vi "MC_Debugging_CreateWireDescription.vi"(6 "End of Interpreted Statement?":bool, 7 "First Error Wire?":bool, 8 "UID?":bool, 9 "Text of Line":string, 10 "Breakpoint Line Numbers":i32[](array[numeric]), 11 "Variable Wire Info":T1) -> (3 "Wire Description":string)   [LabVIEW 2021]
uses:
  <vilib>/imath/engines/lvmath2/MathScriptCompiler/Debugging/MC_Debugging_VariableWireInfo.ctl
  <vilib>/imath/engines/lvmath2/MathScriptCompiler/Debugging/NIMS_Debugging_VariablesCluster.ctl
  <vilib>/imath/engines/lvmath2/RunTimeEngine/Debugging/MC_Debugging_ColVectorInfo.ctl
  <vilib>/imath/engines/lvmath2/RunTimeEngine/Debugging/MC_Debugging_WireData.ctl
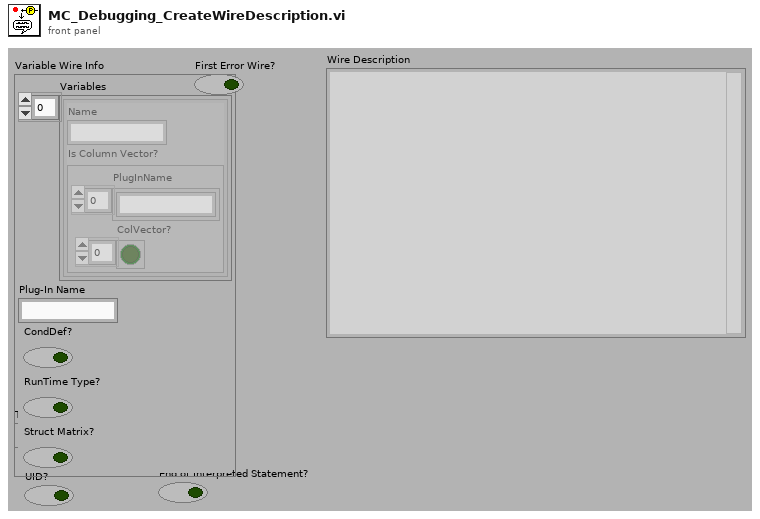
[diagram p1: front panel]
types:
  T1 = typedef "MC_Debugging_VariableWireInfo.ctl" = cluster{"Variables":T2[], "Plug-In Name":string, "CondDef?":bool, "RunTime Type?":bool, "Struct Matrix?":bool}
  T2 = typedef "NIMS_Debugging_VariablesCluster.ctl" = cluster{"Name":string, "Is Column Vector?":T3}
  T3 = typedef "MC_Debugging_ColVectorInfo.ctl" = cluster{"PlugInName":string[], "ColVector?":bool[]}
  T4 = typedef "MC_Debugging_WireData.ctl" = cluster{"Breakpoint Line Numbers":i32[], "Text of Line":string, "UID?":bool, "End of Interpreted Statement?":bool, "Variable Wire Info":T1, "First Error Wire?":bool}
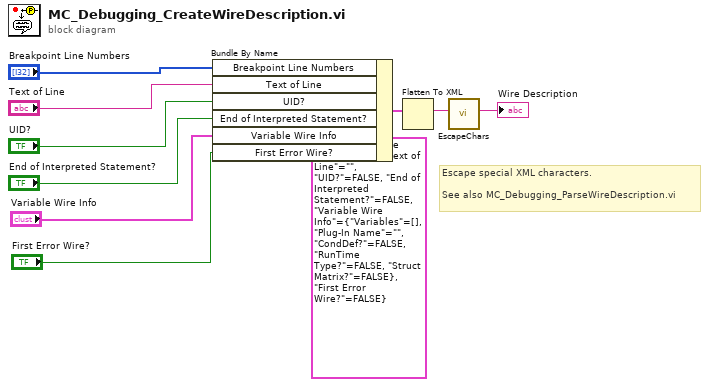
[diagram p0: block diagram]
diagram:
  # "Escape special XML characters.\n\nSee also MC_Debugging_ParseWireDescription.vi"
  n1 = Bundle By Name(cluster=T4 {"Breakpoint Line Numbers"=[], "Text of Line"="", "UID?"=FALSE, "End of Interpreted Statement?"=FALSE, "Variable Wire Info"={"Variables"=[], "Plug-In Name"="", "CondDef?"=FALSE, "RunTime Type?"=FALSE, "Struct Matrix?"=FALSE}, "First Error Wire?"=FALSE} ("Wire Data"), "Breakpoint Line Numbers"="Breakpoint Line Numbers", "Text of Line"="Text of Line", "UID?"="UID?", "End of Interpreted Statement?"="End of Interpreted Statement?", "Variable Wire Info"="Variable Wire Info", "First Error Wire?"="First Error Wire?") -> (w8:T4)
  n2 = Flatten To XML(6:w8) -> (2:w3:string)
  n3 = call <vilib>:"EscapeChars.vi"("XML In"=w3) -> ("XML Out"=→"Wire Description":string)  [unwired: 10 out]
